vi "Type Cast.vi"(0 "image in":refnum<class "MSC Image.lvclass">, 1 "Image Type":T1 items=["Grayscale U8"=0, "Grayscale U16"=2, "Grayscale Single"=5, "Grayscale Double"=6, "RGB U8"=16], 2 "Scale?":bool=TRUE, 5 "error in (no error)":errorcluster) -> (14 "image out":refnum<class "MSC Image.lvclass">, 19 "error out":errorcluster)   [LabVIEW 2014, in "MSC Image.lvclass"]
doc: "Converts the image to the selected type with optional scaling."
uses:
  MSC Image.lvclass
  controls/Image Type.ctl
  MSC Image.lvclass/MSC Image.ctl
  Dependencies/x86/MSC I Process32.dll
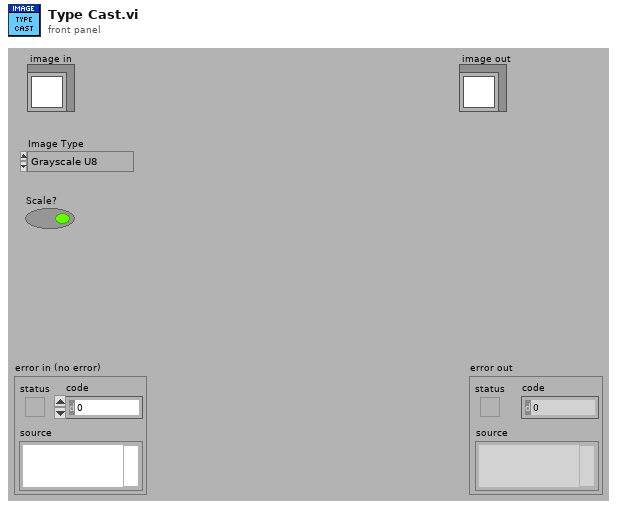
[diagram p1: front panel]
types:
  T1 = typedef "MSC Image.lvclass/Image Type.ctl" = i32
  T2 = typedef "Image.ctl" = cluster{"Pointer":u64, "Size":T3, "Image Type":T4, "Time Stamp":timestamp, "Variant":variant}
  T3 = typedef "Size.ctl" = cluster{"Cols":i32, "Rows":i32}
  T4 = typedef "Image Type.ctl" = i32
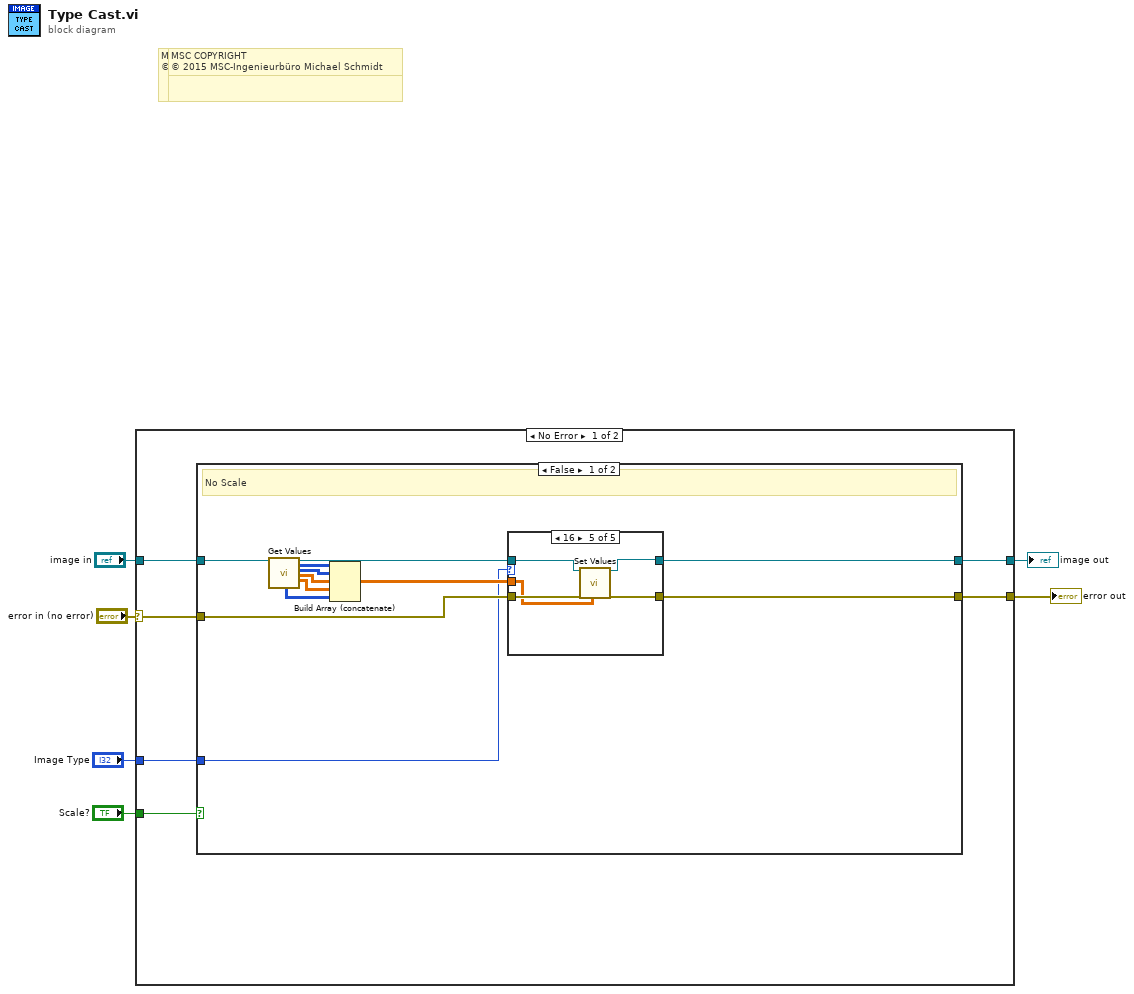
[diagram p0: block diagram]
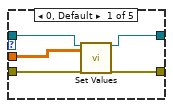
[diagram p2: hidden frame]
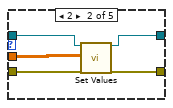
[diagram p3: hidden frame]
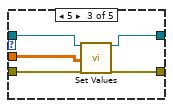
[diagram p4: hidden frame]
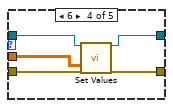
[diagram p5: hidden frame]
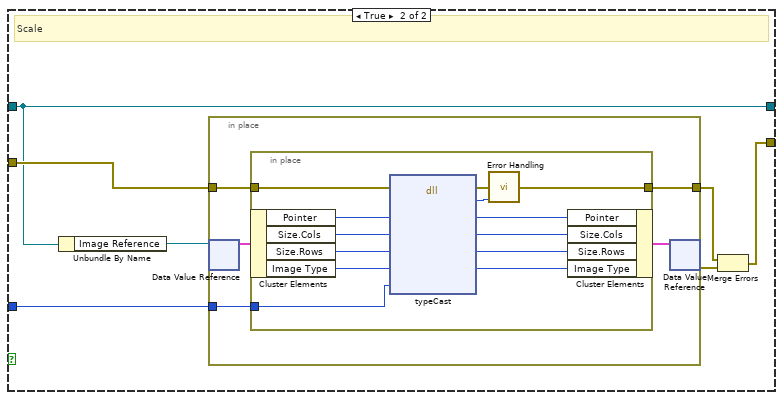
[diagram p6: hidden frame]
diagram:
  # "MSC COPYRIGHT\n© 2016 MSC-Ingenieurbüro Michael Schmidt"
  # "MSC COPYRIGHT\n© 2016 MSC-Ingenieurbüro Michael Schmidt"
  # "MSC COPYRIGHT\n© 2015 MSC-Ingenieurbüro Michael Schmidt"
  # "MSC COPYRIGHT\n© 2015 MSC-Ingenieurbüro Michael Schmidt"
  n1 = case shown="No Error" "error in (no error)" {
    selector: "error in (no error)" -> [w9 w76]
    tunnel: [w8 w76] -> w5
    tunnel: [w7 w75] -> w3
    tunnel: "image in" -> [w10 w75]
    tunnel: "Scale?" -> [w12 _]
    tunnel: "Image Type" -> [w11 _]
    frame No Error {
      n2 = case shown="False" w12 {
        tunnel: [w23 w54] -> w8
        tunnel: w11 -> [w21 w53]
        tunnel: w10 -> [w14 w50]
        tunnel: w9 -> [w24 w51]
        tunnel: [w20 w50] -> w7
        frame False {
          # "No Scale"
          n3 = call-dynamic "Get Values.vi"("image in"=w14) -> ("imageData BGR"=w15:u32[][], "image out"=w13:refnum<class "MSC Image.lvclass">, "imageData U8"=w19:u8[][], "imageData U16"=w18:u16[][], "imageData Single"=w17:sgl[][], "imageData Double"=w16:dbl[][])  [unwired: 11 in, 2 out]
          n4 = Build Array (concatenate)(w19, w18, w17, w16, w15) -> (w22:dbl[][])
          n5 = case shown="16" w21 {
            tunnel: w24 -> [w29 w34 w39 w44 w49]
            tunnel: [w28 w33 w38 w43 w48] -> w23
            tunnel: w22 -> [w27 w30 w35 w40 w45]
            tunnel: w13 -> [w26 w32 w37 w42 w47]
            tunnel: [w25 w31 w36 w41 w46] -> w20
            frame 0, Default {
              n6 = call-dynamic "Set Values.vi"("image in"=w26, "imageData U8"=w27, "error in (no error)"=w29) -> ("image out"=w25:refnum<class "MSC Image.lvclass">, "error out"=w28:errorcluster)  [unwired: 15 in]
            }
            frame 2 {
              n7 = call-dynamic "Set Values.vi"("image in"=w32, "imageData U16"=w30, "error in (no error)"=w34) -> ("image out"=w31:refnum<class "MSC Image.lvclass">, "error out"=w33:errorcluster)  [unwired: 15 in]
            }
            frame 5 {
              n8 = call-dynamic "Set Values.vi"("image in"=w37, "imageData Single"=w35, "error in (no error)"=w39) -> ("image out"=w36:refnum<class "MSC Image.lvclass">, "error out"=w38:errorcluster)  [unwired: 15 in]
            }
            frame 6 {
              n9 = call-dynamic "Set Values.vi"("image in"=w42, "imageData Double"=w40, "error in (no error)"=w44) -> ("image out"=w41:refnum<class "MSC Image.lvclass">, "error out"=w43:errorcluster)  [unwired: 15 in]
            }
            frame 16 {
              n10 = call-dynamic "Set Values.vi"("image in"=w47, "error in (no error)"=w49, "imageData BGR"=w45) -> ("image out"=w46:refnum<class "MSC Image.lvclass">, "error out"=w48:errorcluster)  [unwired: 15 in]
            }
          }
        }
        frame True {
          # "Scale"
          n11 = Unbundle By Name(w50) -> ("Image Reference"=w52:refnum<data-value>)
          n12 = in-place {
            in-place-border: w51 -> [w59]
            in-place-border: [w58] -> w56
            in-place-border: w53 -> [w57]
            n13 = in-place-dvr #1(w52) -> (w60:T2)  [unwired: 1 out]
            n14 = in-place {
              in-place-border: w59 -> [w65]
              in-place-border: [w64] -> w58
              in-place-border: w57 -> [w68]
              n15 = in-place-cluster #2(w60) -> ("Pointer"=w72:u64, "Size.Cols"=w70:i32, "Size.Rows"=w69:i32, "Image Type"=w71:T4)
              n16 = dll-call lib="C:/Users/MSC/LabVIEW Projekte/LV 2014/MSC I-Process/user.lib/MSC-I Process/Dependencies/x86/MSC I Process*.dll" fn="typeCast"(error in=w65, "pointer"=w72, "cols"=w70, "rows"=w69, "type"=w71, "typeTo"=w68) -> (error out=w74:errorcluster, "error"=w73:i32, "pointer"=w63:u64, "cols"=w62:i32, "rows"=w66:i32, "type"=w67:i32)  [unwired: 3 in, 1 out]
              n17 = call "Error Handling.vi"("error in (no error)"=w74, "return type"=w73) -> ("error out"=w64:errorcluster)  [unwired: 12 in, 1 out]
              n18 = in-place-cluster #2("Pointer"=w63, "Size.Cols"=w62, "Size.Rows"=w66, "Image Type"=w67) -> (w61:T2)
            }
            n19 = in-place-dvr #1(w61) -> (w55:errorcluster)  [unwired: 1 out]
          }
          n20 = Merge Errors(w56, w55) -> (w54:errorcluster)
        }
      }
    }
    frame Error {
    }
  }
  "error out" <- w5
  "image out" <- w3
